vi "Parse VI XML - Splitter Size.vi"(8 "Is Vertical?":bool, 9 "UID":i32=83, 10 "New Size":i32, 11 "VI XML":string="<SL__rootObject class=\"oHExt\" uid=\"1\">\n  <root class=\"supC\" uid=\"10\">\n    <objFlags>65536</objFlags>\n    <bounds>(0, 0, 0, 0)</bounds>\n    <MouseWheelSupport>0</MouseWheelSupport>\n    <ddoList elements=\"1\">\n      <SL__arrayElement uid=\"206\"/>\n      </ddoList>\n    <paneHierarchy class=\"splitter\" uid=\"83\">\n      <objFlags>393232</objFlags>\n      <bounds>(46, 0, 434, 621)</bounds>\n      <partsList elements=\"3\">\n        <SL__arrayElement class=\"label\" uid=\"90\">\n          <objFlags>1511754</objFlags>\n          <partID>16</partID>\n          <masterPart>102</masterPart>\n          <howGrow>4108</howGrow>\n          <bounds>(133, 231, 255, 241)</bounds>\n          <image class=\"Image\">\n            <ImageResID>-9</ImageResID>\n            </image>\n          <fgColor>01000000</fgColor>\n          <bgColor>01000000</bgColor>\n          <textRec class=\"textHair\">\n            <mode>1029</mode>\n            <text>\"Splitter\"</text>\n            <bgColor>01000000</bgColor>\n            </textRec>\n          </SL__arrayElement>\n        <SL__arrayElement class=\"bigMultiCosm\" uid=\"91\">\n          <objFlags>2320</objFlags>\n          <partID>102</partID>\n          <bounds>(0, 228, 388, 234)</bounds>\n          <fgColor>00BCBCBC</fgColor>\n          <bgColor>00BCBCBC</bgColor>\n          <index>1</index>\n          <table elements=\"3\">\n            <SL__arrayElement class=\"SubCosm\">\n              <Bounds>(0, 0, 388, 6)</Bounds>\n              <FGColor>00BCBCBC</FGColor>\n              <BGColor>00BCBCBC</BGColor>\n              <Image class=\"Image\">\n                <ImageResID>-428</ImageResID>\n                </Image>\n              </SL__arrayElement>\n            <SL__arrayElement class=\"SubCosm\">\n              <Bounds>(0, 0, 388, 6)</Bounds>\n              <FGColor>00BCBCBC</FGColor>\n              <BGColor>00BCBCBC</BGColor>\n              <Image class=\"Image\">\n                <ImageResID>-11</ImageResID>\n                </Image>\n              </SL__arrayElement>\n            <SL__arrayElement class=\"SubCosm\">\n              <Bounds>(0, 0, 388, 6)</Bounds>\n              <FGColor>01000016</FGColor>\n              <BGColor>01000016</BGColor>\n              <Image class=\"Image\">\n                <ImageResID>-9</ImageResID>\n                </Image>\n              </SL__arrayElement>\n            </table>\n          </SL__arrayElement>\n        <SL__arrayElement class=\"annex\" uid=\"92\">\n          <partID>66</partID>\n          <refListLength>0</refListLength>\n          <hGrowNodeListLength>1</hGrowNodeListLength>\n          </SL__arrayElement>\n        </partsList>\n      <topOrLeft class=\"pane\" uid=\"104\">\n        <objFlags>2492464</objFlags>\n        <bounds>(0, 0, 388, 228)</bounds>\n        <partsList elements=\"6\">\n          <SL__arrayElement class=\"label\" uid=\"107\">\n            <objFlags>1511754</objFlags>\n            <partID>16</partID>\n            <masterPart>28</masterPart>\n            <howGrow>5</howGrow>\n            <bounds>(0, 0, 17, 29)</bounds>\n            <image class=\"Image\">\n              <ImageResID>-9</ImageResID>\n              </image>\n            <fgColor>01000000</fgColor>\n            <bgColor>01000000</bgColor>\n            <textRec class=\"textHair\">\n              <mode>1028</mode>\n              <text>\"Pane\"</text>\n              <bgColor>01000000</bgColor>\n              </textRec>\n            </SL__arrayElement>\n          <SL__arrayElement class=\"cosm\" uid=\"108\">\n            <objFlags>3442</objFlags>\n            <partID>39</partID>\n            <masterPart>28</masterPart>\n            <howGrow>194</howGrow>\n            <bounds>(0, 211, 371, 228)</bounds>\n            <image class=\"Image\">\n              <ImageResID>0</ImageResID>\n              </image>\n            <bgColor>00B3B3B3</bgColor>\n            </SL__arrayElement>\n          <SL__arrayElement class=\"cosm\" uid=\"109\">\n            <objFlags>3442</objFlags>\n            <partID>38</partID>\n            <masterPart>28</masterPart>\n            <howGrow>56</howGrow>\n            <bounds>(371, 0, 388, 211)</bounds>\n            <image class=\"Image\">\n              <ImageResID>0</ImageResID>\n              </image>\n            <bgColor>00B3B3B3</bgColor>\n            </SL__arrayElement>\n          <SL__arrayElement class=\"cosm\" uid=\"110\">\n            <objFlags>3443</objFlags>\n            <partID>44</partID>\n            <masterPart>28</masterPart>\n            <howGrow>10</howGrow>\n            <bounds>(371, 211, 388, 228)</bounds>\n            <image class=\"Image\">\n              <ImageResID>-365</ImageResID>\n              </image>\n            <fgColor>00B3B3B3</fgColor>\n            <bgColor>00B3B3B3</bgColor>\n            </SL__arrayElement>\n          <SL__arrayElement class=\"cosm\" uid=\"111\">\n            <objFlags>115</objFlags>\n            <partID>28</partID>\n            <howGrow>120</howGrow>\n            <bounds>(0, 0, 371, 211)</bounds>\n            <image class=\"Image\">\n              <ImageResID>-704</ImageResID>\n              </image>\n            <fgColor>00E2E2E2</fgColor>\n            <bgColor>00E2E2E2</bgColor>\n            </SL__arrayElement>\n          <SL__arrayElement class=\"annex\" uid=\"112\">\n            <partID>66</partID>\n            </SL__arrayElement>\n          </partsList>\n        <paneFlags>331089</paneFlags>\n        <minPaneSize>(1,1)</minPaneSize>\n        <docBounds>(-138, 0, 325, 232)</docBounds>\n        <zPlaneList elements=\"1\">\n          <SL__arrayElement class=\"fPDCO\" uid=\"206\">\n            <objFlags>1</objFlags>\n            <typeDesc>TypeID(1)</typeDesc>\n            <ddo class=\"stdNum\" uid=\"190\">\n              <objFlags>393217</objFlags>\n              <bounds>(0, 105, 41, 180)</bounds>\n              <partsList elements=\"8\">\n                <SL__arrayElement class=\"label\" uid=\"196\">\n                  <objFlags>1507654</objFlags>\n                  <partID>16</partID>\n                  <masterPart>9</masterPart>\n                  <howGrow>4096</howGrow>\n                  <bounds>(0, 0, 17, 22)</bounds>\n                  <image class=\"Image\">\n                    <ImageResID>-9</ImageResID>\n                    </image>\n                  <fgColor>01000000</fgColor>\n                  <bgColor>01000000</bgColor>\n                  <textRec class=\"textHair\">\n                    <flags>512</flags>\n                    <mode>17412</mode>\n                    <text>\"UID\"</text>\n                    <bgColor>01000000</bgColor>\n                    </textRec>\n                  </SL__arrayElement>\n                <SL__arrayElement class=\"numLabel\" uid=\"197\">\n                  <objFlags>264498</objFlags>\n                  <partID>10</partID>\n                  <masterPart>9</masterPart>\n                  <howGrow>240</howGrow>\n                  <bounds>(19, 2, 39, 74)</bounds>\n                  <image class=\"Image\">\n                    <ImageResID>-2002</ImageResID>\n                    </image>\n                  <fgColor>00FFFFFF</fgColor>\n                  <bgColor>00E8EBED</bgColor>\n                  <textRec class=\"textHair\">\n                    <flags>1536</flags>\n                    <mode>8389650</mode>\n                    <view>(1, 0, -2, 0)</view>\n                    <bgColor>00E8EBED</bgColor>\n                    </textRec>\n                  <format>\"%25.0f\"</format>\n                  </SL__arrayElement>\n                <SL__arrayElement class=\"bigMultiCosm\" uid=\"198\">\n                  <objFlags>6458</objFlags>\n                  <partID>2</partID>\n                  <masterPart>9</masterPart>\n                  <howGrow>2054</howGrow>\n                  <bounds>(17, 62, 28, 75)</bounds>\n                  <fgColor>002B3033</fgColor>\n                  <bgColor>00A8ABAE</bgColor>\n                  <table elements=\"2\">\n                    <SL__arrayElement class=\"SubCosm\">\n                      <Bounds>(0, 0, 11, 13)</Bounds>\n                      <FGColor>002B3033</FGColor>\n                      <BGColor>00A8ABAE</BGColor>\n                      <Image class=\"Image\">\n                        <ImageResID>-774</ImageResID>\n                        </Image>\n                      </SL__arrayElement>\n                    <SL__arrayElement class=\"SubCosm\">\n                      <Bounds>(0, 0, 11, 13)</Bounds>\n                      <FGColor>002B3033</FGColor>\n                      <BGColor>004384B7</BGColor>\n                      <Image class=\"Image\">\n                        <ImageResID>-774</ImageResID>\n                        </Image>\n                      </SL__arrayElement>\n                    </table>\n                  </SL__arrayElement>\n                <SL__arrayElement class=\"bigMultiCosm\" uid=\"199\">\n                  <objFlags>6458</objFlags>\n                  <partID>3</partID>\n                  <masterPart>9</masterPart>\n                  <howGrow>1034</howGrow>\n                  <bounds>(30, 62, 41, 75)</bounds>\n                  <fgColor>002B3033</fgColor>\n                  <bgColor>00A8ABAE</bgColor>\n                  <table elements=\"2\">\n                    <SL__arrayElement class=\"SubCosm\">\n                      <Bounds>(0, 0, 11, 13)</Bounds>\n                      <FGColor>002B3033</FGColor>\n                      <BGColor>00A8ABAE</BGColor>\n                      <Image class=\"Image\">\n                        <ImageResID>-775</ImageResID>\n                        </Image>\n                      </SL__arrayElement>\n                    <SL__arrayElement class=\"SubCosm\">\n                      <Bounds>(0, 0, 11, 13)</Bounds>\n                      <FGColor>002B3033</FGColor>\n                      <BGColor>004384B7</BGColor>\n                      <Image class=\"Image\">\n                        <ImageResID>-775</ImageResID>\n                        </Image>\n                      </SL__arrayElement>\n                    </table>\n                  </SL__arrayElement>\n                <SL__arrayElement class=\"multiCosm\" uid=\"200\">\n                  <objFlags>6458</objFlags>\n                  <partID>15</partID>\n                  <masterPart>9</masterPart>\n                  <howGrow>13</howGrow>\n                  <bounds>(22, 1, 37, 7)</bounds>\n                  <fgColor>002B3033</fgColor>\n                  <bgColor>00DBDFE2</bgColor>\n                  <table elements=\"5\">\n                    <SL__arrayElement class=\"Image\">\n                      <ImageResID>-2000</ImageResID>\n                      </SL__arrayElement>\n                    <SL__arrayElement class=\"Image\">\n                      <ImageResID>-2001</ImageResID>\n                      </SL__arrayElement>\n                    <SL__arrayElement class=\"Image\">\n                      <ImageResID>-2002</ImageResID>\n                      </SL__arrayElement>\n                    <SL__arrayElement class=\"Image\">\n                      <ImageResID>-2003</ImageResID>\n                      </SL__arrayElement>\n                    <SL__arrayElement class=\"Image\">\n                      <ImageResID>-2095</ImageResID>\n                      </SL__arrayElement>\n                    </table>\n                  </SL__arrayElement>\n                <SL__arrayElement class=\"multiCosm\" uid=\"201\">\n                  <objFlags>6462</objFlags>\n                  <partID>118</partID>\n                  <masterPart>9</masterPart>\n                  <howGrow>193</howGrow>\n                  <bounds>(18, 1, 40, 7)</bounds>\n                  <fgColor>00DBDFE2</fgColor>\n                  <bgColor>00DBDFE2</bgColor>\n                  <table elements=\"5\">\n                    <SL__arrayElement class=\"Image\">\n                      <ImageResID>-11</ImageResID>\n                      </SL__arrayElement>\n                    <SL__arrayElement class=\"Image\">\n                      <ImageResID>-11</ImageResID>\n                      </SL__arrayElement>\n                    <SL__arrayElement class=\"Image\">\n                      <ImageResID>-11</ImageResID>\n                      </SL__arrayElement>\n                    <SL__arrayElement class=\"Image\">\n                      <ImageResID>-11</ImageResID>\n                      </SL__arrayElement>\n                    <SL__arrayElement class=\"Image\">\n                      <ImageResID>-11</ImageResID>\n                      </SL__arrayElement>\n                    </table>\n                  </SL__arrayElement>\n                <SL__arrayElement class=\"cosm\" uid=\"202\">\n                  <objFlags>2327</objFlags>\n                  <partID>9</partID>\n                  <howGrow>240</howGrow>\n                  <bounds>(17, 0, 41, 75)</bounds>\n                  <image class=\"Image\">\n                    <ImageResID>-786</ImageResID>\n                    </image>\n                  <fgColor>00A8ABAE</fgColor>\n                  <bgColor>00E8EBED</bgColor>\n                  </SL__arrayElement>\n                <SL__arrayElement class=\"annex\" uid=\"203\">\n                  <partID>66</partID>\n                  <refListLength>0</refListLength>\n                  <hGrowNodeListLength>0</hGrowNodeListLength>\n                  <rsrcID>32707</rsrcID>\n                  </SL__arrayElement>\n                </partsList>\n              <typeDesc>TypeID(2)</typeDesc>\n              <MouseWheelSupport>2</MouseWheelSupport>\n              <StdNumMin>-2147483648</StdNumMin>\n              <StdNumMax>2147483647</StdNumMax>\n              <StdNumInc>0</StdNumInc>\n              </ddo>\n            <conNum>-1</conNum>\n            <termListLength>1</termListLength>\n            </SL__arrayElement>\n          </zPlaneList>\n        <image class=\"Image\">\n          <ImageResID>0</ImageResID>\n          </image>\n        </topOrLeft>\n      <botOrRight class=\"pane\" uid=\"95\">\n        <objFlags>2492464</objFlags>\n        <bounds>(0, 234, 388, 621)</bounds>\n        <partsList elements=\"6\">\n          <SL__arrayElement class=\"label\" uid=\"98\">\n            <objFlags>1511754</objFlags>\n            <partID>16</partID>\n            <masterPart>28</masterPart>\n            <howGrow>5</howGrow>\n            <bounds>(0, 0, 17, 38)</bounds>\n            <image class=\"Image\">\n              <ImageResID>-9</ImageResID>\n              </image>\n            <fgColor>01000000</fgColor>\n            <bgColor>01000000</bgColor>\n            <textRec class=\"textHair\">\n              <mode>1028</mode>\n              <text>\"Pane 2\"</text>\n              <bgColor>01000000</bgColor>\n              </textRec>\n            </SL__arrayElement>\n          <SL__arrayElement class=\"cosm\" uid=\"99\">\n            <objFlags>3442</objFlags>\n            <partID>39</partID>\n            <masterPart>28</masterPart>\n            <howGrow>194</howGrow>\n            <bounds>(0, 370, 371, 387)</bounds>\n            <image class=\"Image\">\n              <ImageResID>0</ImageResID>\n              </image>\n            <bgColor>00B3B3B3</bgColor>\n            </SL__arrayElement>\n          <SL__arrayElement class=\"cosm\" uid=\"100\">\n            <objFlags>3442</objFlags>\n            <partID>38</partID>\n            <masterPart>28</masterPart>\n            <howGrow>56</howGrow>\n            <bounds>(371, 0, 388, 370)</bounds>\n            <image class=\"Image\">\n              <ImageResID>0</ImageResID>\n              </image>\n            <bgColor>00B3B3B3</bgColor>\n            </SL__arrayElement>\n          <SL__arrayElement class=\"cosm\" uid=\"101\">\n            <objFlags>3443</objFlags>\n            <partID>44</partID>\n            <masterPart>28</masterPart>\n            <howGrow>10</howGrow>\n            <bounds>(371, 370, 388, 387)</bounds>\n            <image class=\"Image\">\n              <ImageResID>-365</ImageResID>\n              </image>\n            <fgColor>00B3B3B3</fgColor>\n            <bgColor>00B3B3B3</bgColor>\n            </SL__arrayElement>\n          <SL__arrayElement class=\"cosm\" uid=\"102\">\n            <objFlags>115</objFlags>\n            <partID>28</partID>\n            <howGrow>120</howGrow>\n            <bounds>(0, 0, 371, 370)</bounds>\n            <image class=\"Image\">\n              <ImageResID>-704</ImageResID>\n              </image>\n            <fgColor>00E2E2E2</fgColor>\n            <bgColor>00E2E2E2</bgColor>\n            </SL__arrayElement>\n          <SL__arrayElement class=\"annex\" uid=\"103\">\n            <partID>66</partID>\n            </SL__arrayElement>\n          </partsList>\n        <paneFlags>331089</paneFlags>\n        <minPaneSize>(1,1)</minPaneSize>\n        <docBounds>(-46, 0, 325, 370)</docBounds>\n        <zPlaneList elements=\"0\">\n          </zPlaneList>\n        <image class=\"Image\">\n          <ImageResID>0</ImageResID>\n          </image>\n        </botOrRight>\n      <splitterFlags>1</splitterFlags>\n      <ratio>3.671498E-1 (%x0EFBBB3E)</ratio>\n      </paneHierarchy>\n    <savedSize>(0, 0, 0, 0)</savedSize>\n    <conPane class=\"conPane\" uid=\"21\">\n      <conId>4815</conId>\n      <cons elements=\"12\">\n        </cons>\n      </conPane>\n    <keyMappingList class=\"keyMapList\" uid=\"22\">\n      </keyMappingList>\n    </root>\n  <pBounds>(46, 0, 434, 621)</pBounds>\n  <dBounds>(0, 0, 0, 0)</dBounds>\n  <origin>(435,189)</origin>\n  <instrStyle>31</instrStyle>\n  <blinkList elements=\"0\">\n    </blinkList>\n  </SL__rootObject>\n") -> (2 "Old Size":i32, 3 "VI XML With New Size":string="<SL__rootObject class=\"oHExt\" uid=\"1\">\n  <root class=\"supC\" uid=\"10\">\n    <objFlags>65536</objFlags>\n    <bounds>(0, 0, 0, 0)</bounds>\n    <MouseWheelSupport>0</MouseWheelSupport>\n    <ddoList elements=\"1\">\n      <SL__arrayElement uid=\"206\"/>\n      </ddoList>\n    <paneHierarchy class=\"splitter\" uid=\"83\">\n      <objFlags>393232</objFlags>\n      <bounds>(46, 0, 434, 621)</bounds>\n      <partsList elements=\"3\">\n        <SL__arrayElement class=\"label\" uid=\"90\">\n          <objFlags>1511754</objFlags>\n          <partID>16</partID>\n          <masterPart>102</masterPart>\n          <howGrow>4108</howGrow>\n          <bounds>(133, 231, 255, 241)</bounds>\n          <image class=\"Image\">\n            <ImageResID>-9</ImageResID>\n            </image>\n          <fgColor>01000000</fgColor>\n          <bgColor>01000000</bgColor>\n          <textRec class=\"textHair\">\n            <mode>1029</mode>\n            <text>\"Splitter\"</text>\n            <bgColor>01000000</bgColor>\n            </textRec>\n          </SL__arrayElement>\n        <SL__arrayElement class=\"bigMultiCosm\" uid=\"91\">\n          <objFlags>2320</objFlags>\n          <partID>102</partID>\n          <bounds>(0, 228, 388, 234)</bounds>\n          <fgColor>00BCBCBC</fgColor>\n          <bgColor>00BCBCBC</bgColor>\n          <index>1</index>\n          <table elements=\"3\">\n            <SL__arrayElement class=\"SubCosm\">\n              <Bounds>(0, 0, 388, 6)</Bounds>\n              <FGColor>00BCBCBC</FGColor>\n              <BGColor>00BCBCBC</BGColor>\n              <Image class=\"Image\">\n                <ImageResID>-428</ImageResID>\n                </Image>\n              </SL__arrayElement>\n            <SL__arrayElement class=\"SubCosm\">\n              <Bounds>(0, 0, 388, 6)</Bounds>\n              <FGColor>00BCBCBC</FGColor>\n              <BGColor>00BCBCBC</BGColor>\n              <Image class=\"Image\">\n                <ImageResID>-11</ImageResID>\n                </Image>\n              </SL__arrayElement>\n            <SL__arrayElement class=\"SubCosm\">\n              <Bounds>(0, 0, 388, 6)</Bounds>\n              <FGColor>01000016</FGColor>\n              <BGColor>01000016</BGColor>\n              <Image class=\"Image\">\n                <ImageResID>-9</ImageResID>\n                </Image>\n              </SL__arrayElement>\n            </table>\n          </SL__arrayElement>\n        <SL__arrayElement class=\"annex\" uid=\"92\">\n          <partID>66</partID>\n          <refListLength>0</refListLength>\n          <hGrowNodeListLength>1</hGrowNodeListLength>\n          </SL__arrayElement>\n        </partsList>\n      <topOrLeft class=\"pane\" uid=\"104\">\n        <objFlags>2492464</objFlags>\n        <bounds>(0, 0, 388, 228)</bounds>\n        <partsList elements=\"6\">\n          <SL__arrayElement class=\"label\" uid=\"107\">\n            <objFlags>1511754</objFlags>\n            <partID>16</partID>\n            <masterPart>28</masterPart>\n            <howGrow>5</howGrow>\n            <bounds>(0, 0, 17, 29)</bounds>\n            <image class=\"Image\">\n              <ImageResID>-9</ImageResID>\n              </image>\n            <fgColor>01000000</fgColor>\n            <bgColor>01000000</bgColor>\n            <textRec class=\"textHair\">\n              <mode>1028</mode>\n              <text>\"Pane\"</text>\n              <bgColor>01000000</bgColor>\n              </textRec>\n            </SL__arrayElement>\n          <SL__arrayElement class=\"cosm\" uid=\"108\">\n            <objFlags>3442</objFlags>\n            <partID>39</partID>\n            <masterPart>28</masterPart>\n            <howGrow>194</howGrow>\n            <bounds>(0, 211, 371, 228)</bounds>\n            <image class=\"Image\">\n              <ImageResID>0</ImageResID>\n              </image>\n            <bgColor>00B3B3B3</bgColor>\n            </SL__arrayElement>\n          <SL__arrayElement class=\"cosm\" uid=\"109\">\n            <objFlags>3442</objFlags>\n            <partID>38</partID>\n            <masterPart>28</masterPart>\n            <howGrow>56</howGrow>\n            <bounds>(371, 0, 388, 211)</bounds>\n            <image class=\"Image\">\n              <ImageResID>0</ImageResID>\n              </image>\n            <bgColor>00B3B3B3</bgColor>\n            </SL__arrayElement>\n          <SL__arrayElement class=\"cosm\" uid=\"110\">\n            <objFlags>3443</objFlags>\n            <partID>44</partID>\n            <masterPart>28</masterPart>\n            <howGrow>10</howGrow>\n            <bounds>(371, 211, 388, 228)</bounds>\n            <image class=\"Image\">\n              <ImageResID>-365</ImageResID>\n              </image>\n            <fgColor>00B3B3B3</fgColor>\n            <bgColor>00B3B3B3</bgColor>\n            </SL__arrayElement>\n          <SL__arrayElement class=\"cosm\" uid=\"111\">\n            <objFlags>115</objFlags>\n            <partID>28</partID>\n            <howGrow>120</howGrow>\n            <bounds>(0, 0, 371, 211)</bounds>\n            <image class=\"Image\">\n              <ImageResID>-704</ImageResID>\n              </image>\n            <fgColor>00E2E2E2</fgColor>\n            <bgColor>00E2E2E2</bgColor>\n            </SL__arrayElement>\n          <SL__arrayElement class=\"annex\" uid=\"112\">\n            <partID>66</partID>\n            </SL__arrayElement>\n          </partsList>\n        <paneFlags>331089</paneFlags>\n        <minPaneSize>(1,1)</minPaneSize>\n        <docBounds>(-138, 0, 325, 232)</docBounds>\n        <zPlaneList elements=\"1\">\n          <SL__arrayElement class=\"fPDCO\" uid=\"206\">\n            <objFlags>1</objFlags>\n            <typeDesc>TypeID(1)</typeDesc>\n            <ddo class=\"stdNum\" uid=\"190\">\n              <objFlags>393217</objFlags>\n              <bounds>(0, 105, 41, 180)</bounds>\n              <partsList elements=\"8\">\n                <SL__arrayElement class=\"label\" uid=\"196\">\n                  <objFlags>1507654</objFlags>\n                  <partID>16</partID>\n                  <masterPart>9</masterPart>\n                  <howGrow>4096</howGrow>\n                  <bounds>(0, 0, 17, 22)</bounds>\n                  <image class=\"Image\">\n                    <ImageResID>-9</ImageResID>\n                    </image>\n                  <fgColor>01000000</fgColor>\n                  <bgColor>01000000</bgColor>\n                  <textRec class=\"textHair\">\n                    <flags>512</flags>\n                    <mode>17412</mode>\n                    <text>\"UID\"</text>\n                    <bgColor>01000000</bgColor>\n                    </textRec>\n                  </SL__arrayElement>\n                <SL__arrayElement class=\"numLabel\" uid=\"197\">\n                  <objFlags>264498</objFlags>\n                  <partID>10</partID>\n                  <masterPart>9</masterPart>\n                  <howGrow>240</howGrow>\n                  <bounds>(19, 2, 39, 74)</bounds>\n                  <image class=\"Image\">\n                    <ImageResID>-2002</ImageResID>\n                    </image>\n                  <fgColor>00FFFFFF</fgColor>\n                  <bgColor>00E8EBED</bgColor>\n                  <textRec class=\"textHair\">\n                    <flags>1536</flags>\n                    <mode>8389650</mode>\n                    <view>(1, 0, -2, 0)</view>\n                    <bgColor>00E8EBED</bgColor>\n                    </textRec>\n                  <format>\"%25.0f\"</format>\n                  </SL__arrayElement>\n                <SL__arrayElement class=\"bigMultiCosm\" uid=\"198\">\n                  <objFlags>6458</objFlags>\n                  <partID>2</partID>\n                  <masterPart>9</masterPart>\n                  <howGrow>2054</howGrow>\n                  <bounds>(17, 62, 28, 75)</bounds>\n                  <fgColor>002B3033</fgColor>\n                  <bgColor>00A8ABAE</bgColor>\n                  <table elements=\"2\">\n                    <SL__arrayElement class=\"SubCosm\">\n                      <Bounds>(0, 0, 11, 13)</Bounds>\n                      <FGColor>002B3033</FGColor>\n                      <BGColor>00A8ABAE</BGColor>\n                      <Image class=\"Image\">\n                        <ImageResID>-774</ImageResID>\n                        </Image>\n                      </SL__arrayElement>\n                    <SL__arrayElement class=\"SubCosm\">\n                      <Bounds>(0, 0, 11, 13)</Bounds>\n                      <FGColor>002B3033</FGColor>\n                      <BGColor>004384B7</BGColor>\n                      <Image class=\"Image\">\n                        <ImageResID>-774</ImageResID>\n                        </Image>\n                      </SL__arrayElement>\n                    </table>\n                  </SL__arrayElement>\n                <SL__arrayElement class=\"bigMultiCosm\" uid=\"199\">\n                  <objFlags>6458</objFlags>\n                  <partID>3</partID>\n                  <masterPart>9</masterPart>\n                  <howGrow>1034</howGrow>\n                  <bounds>(30, 62, 41, 75)</bounds>\n                  <fgColor>002B3033</fgColor>\n                  <bgColor>00A8ABAE</bgColor>\n                  <table elements=\"2\">\n                    <SL__arrayElement class=\"SubCosm\">\n                      <Bounds>(0, 0, 11, 13)</Bounds>\n                      <FGColor>002B3033</FGColor>\n                      <BGColor>00A8ABAE</BGColor>\n                      <Image class=\"Image\">\n                        <ImageResID>-775</ImageResID>\n                        </Image>\n                      </SL__arrayElement>\n                    <SL__arrayElement class=\"SubCosm\">\n                      <Bounds>(0, 0, 11, 13)</Bounds>\n                      <FGColor>002B3033</FGColor>\n                      <BGColor>004384B7</BGColor>\n                      <Image class=\"Image\">\n                        <ImageResID>-775</ImageResID>\n                        </Image>\n                      </SL__arrayElement>\n                    </table>\n                  </SL__arrayElement>\n                <SL__arrayElement class=\"multiCosm\" uid=\"200\">\n                  <objFlags>6458</objFlags>\n                  <partID>15</partID>\n                  <masterPart>9</masterPart>\n                  <howGrow>13</howGrow>\n                  <bounds>(22, 1, 37, 7)</bounds>\n                  <fgColor>002B3033</fgColor>\n                  <bgColor>00DBDFE2</bgColor>\n                  <table elements=\"5\">\n                    <SL__arrayElement class=\"Image\">\n                      <ImageResID>-2000</ImageResID>\n                      </SL__arrayElement>\n                    <SL__arrayElement class=\"Image\">\n                      <ImageResID>-2001</ImageResID>\n                      </SL__arrayElement>\n                    <SL__arrayElement class=\"Image\">\n                      <ImageResID>-2002</ImageResID>\n                      </SL__arrayElement>\n                    <SL__arrayElement class=\"Image\">\n                      <ImageResID>-2003</ImageResID>\n                      </SL__arrayElement>\n                    <SL__arrayElement class=\"Image\">\n                      <ImageResID>-2095</ImageResID>\n                      </SL__arrayElement>\n                    </table>\n                  </SL__arrayElement>\n                <SL__arrayElement class=\"multiCosm\" uid=\"201\">\n                  <objFlags>6462</objFlags>\n                  <partID>118</partID>\n                  <masterPart>9</masterPart>\n                  <howGrow>193</howGrow>\n                  <bounds>(18, 1, 40, 7)</bounds>\n                  <fgColor>00DBDFE2</fgColor>\n                  <bgColor>00DBDFE2</bgColor>\n                  <table elements=\"5\">\n                    <SL__arrayElement class=\"Image\">\n                      <ImageResID>-11</ImageResID>\n                      </SL__arrayElement>\n                    <SL__arrayElement class=\"Image\">\n                      <ImageResID>-11</ImageResID>\n                      </SL__arrayElement>\n                    <SL__arrayElement class=\"Image\">\n                      <ImageResID>-11</ImageResID>\n                      </SL__arrayElement>\n                    <SL__arrayElement class=\"Image\">\n                      <ImageResID>-11</ImageResID>\n                      </SL__arrayElement>\n                    <SL__arrayElement class=\"Image\">\n                      <ImageResID>-11</ImageResID>\n                      </SL__arrayElement>\n                    </table>\n                  </SL__arrayElement>\n                <SL__arrayElement class=\"cosm\" uid=\"202\">\n                  <objFlags>2327</objFlags>\n                  <partID>9</partID>\n                  <howGrow>240</howGrow>\n                  <bounds>(17, 0, 41, 75)</bounds>\n                  <image class=\"Image\">\n                    <ImageResID>-786</ImageResID>\n                    </image>\n                  <fgColor>00A8ABAE</fgColor>\n                  <bgColor>00E8EBED</bgColor>\n                  </SL__arrayElement>\n                <SL__arrayElement class=\"annex\" uid=\"203\">\n                  <partID>66</partID>\n                  <refListLength>0</refListLength>\n                  <hGrowNodeListLength>0</hGrowNodeListLength>\n                  <rsrcID>32707</rsrcID>\n                  </SL__arrayElement>\n                </partsList>\n              <typeDesc>TypeID(2)</typeDesc>\n              <MouseWheelSupport>2</MouseWheelSupport>\n              <StdNumMin>-2147483648</StdNumMin>\n              <StdNumMax>2147483647</StdNumMax>\n              <StdNumInc>0</StdNumInc>\n              </ddo>\n            <conNum>-1</conNum>\n            <termListLength>1</termListLength>\n            </SL__arrayElement>\n          </zPlaneList>\n        <image class=\"Image\">\n          <ImageResID>0</ImageResID>\n          </image>\n        </topOrLeft>\n      <botOrRight class=\"pane\" uid=\"95\">\n        <objFlags>2492464</objFlags>\n        <bounds>(0, 234, 388, 621)</bounds>\n        <partsList elements=\"6\">\n          <SL__arrayElement class=\"label\" uid=\"98\">\n            <objFlags>1511754</objFlags>\n            <partID>16</partID>\n            <masterPart>28</masterPart>\n            <howGrow>5</howGrow>\n            <bounds>(0, 0, 17, 38)</bounds>\n            <image class=\"Image\">\n              <ImageResID>-9</ImageResID>\n              </image>\n            <fgColor>01000000</fgColor>\n            <bgColor>01000000</bgColor>\n            <textRec class=\"textHair\">\n              <mode>1028</mode>\n              <text>\"Pane 2\"</text>\n              <bgColor>01000000</bgColor>\n              </textRec>\n            </SL__arrayElement>\n          <SL__arrayElement class=\"cosm\" uid=\"99\">\n            <objFlags>3442</objFlags>\n            <partID>39</partID>\n            <masterPart>28</masterPart>\n            <howGrow>194</howGrow>\n            <bounds>(0, 370, 371, 387)</bounds>\n            <image class=\"Image\">\n              <ImageResID>0</ImageResID>\n              </image>\n            <bgColor>00B3B3B3</bgColor>\n            </SL__arrayElement>\n          <SL__arrayElement class=\"cosm\" uid=\"100\">\n            <objFlags>3442</objFlags>\n            <partID>38</partID>\n            <masterPart>28</masterPart>\n            <howGrow>56</howGrow>\n            <bounds>(371, 0, 388, 370)</bounds>\n            <image class=\"Image\">\n              <ImageResID>0</ImageResID>\n              </image>\n            <bgColor>00B3B3B3</bgColor>\n            </SL__arrayElement>\n          <SL__arrayElement class=\"cosm\" uid=\"101\">\n            <objFlags>3443</objFlags>\n            <partID>44</partID>\n            <masterPart>28</masterPart>\n            <howGrow>10</howGrow>\n            <bounds>(371, 370, 388, 387)</bounds>\n            <image class=\"Image\">\n              <ImageResID>-365</ImageResID>\n              </image>\n            <fgColor>00B3B3B3</fgColor>\n            <bgColor>00B3B3B3</bgColor>\n            </SL__arrayElement>\n          <SL__arrayElement class=\"cosm\" uid=\"102\">\n            <objFlags>115</objFlags>\n            <partID>28</partID>\n            <howGrow>120</howGrow>\n            <bounds>(0, 0, 371, 370)</bounds>\n            <image class=\"Image\">\n              <ImageResID>-704</ImageResID>\n              </image>\n            <fgColor>00E2E2E2</fgColor>\n            <bgColor>00E2E2E2</bgColor>\n            </SL__arrayElement>\n          <SL__arrayElement class=\"annex\" uid=\"103\">\n            <partID>66</partID>\n            </SL__arrayElement>\n          </partsList>\n        <paneFlags>331089</paneFlags>\n        <minPaneSize>(1,1)</minPaneSize>\n        <docBounds>(-46, 0, 325, 370)</docBounds>\n        <zPlaneList elements=\"0\">\n          </zPlaneList>\n        <image class=\"Image\">\n          <ImageResID>0</ImageResID>\n          </image>\n        </botOrRight>\n      <splitterFlags>1</splitterFlags>\n      <ratio>3.671498E-1 (%x0EFBBB3E)</ratio>\n      </paneHierarchy>\n    <savedSize>(0, 0, 0, 0)</savedSize>\n    <conPane class=\"conPane\" uid=\"21\">\n      <conId>4815</conId>\n      <cons elements=\"12\">\n        </cons>\n      </conPane>\n    <keyMappingList class=\"keyMapList\" uid=\"22\">\n      </keyMappingList>\n    </root>\n  <pBounds>(46, 0, 434, 621)</pBounds>\n  <dBounds>(0, 0, 0, 0)</dBounds>\n  <origin>(435,189)</origin>\n  <instrStyle>31</instrStyle>\n  <blinkList elements=\"0\">\n    </blinkList>\n  </SL__rootObject>\n")   [LabVIEW 2015, in "Splitter.lvclass"]
uses:
  Splitter.lvclass
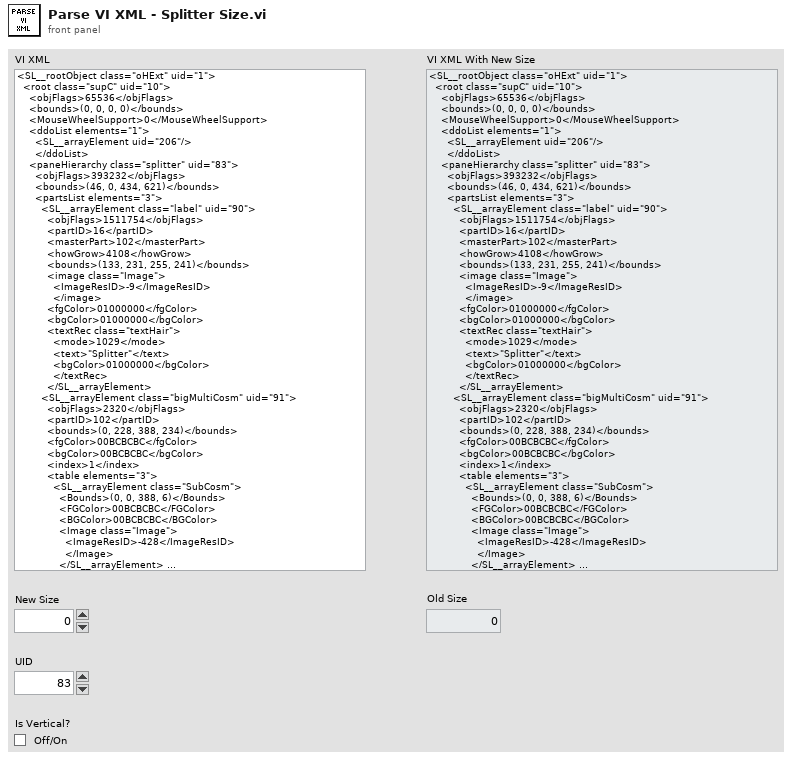
[diagram p1: front panel]
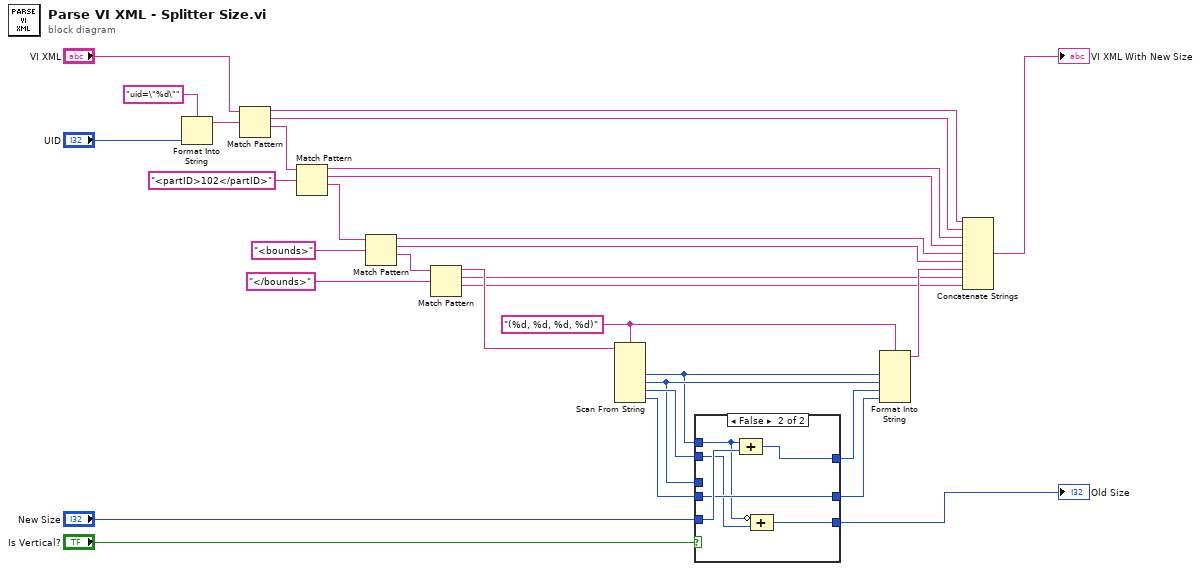
[diagram p0: block diagram]
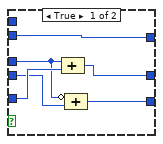
[diagram p2: hidden frame]
diagram:
  w21 = "(%d, %d, %d, %d)" ("format string")
  n1 = Format Into String(format string="uid=\"%d\"", "UID") -> (resulting string=w30:string)  [unwired: 2 in, 1 out]
  n2 = Match Pattern(string="VI XML", regular expression=w30) -> (before substring=w12:string, match substring=w13:string, after substring=w28:string)  [unwired: 1 in, 1 out]
  n3 = Match Pattern(string=w28, regular expression="<partID>102</partID>" ("format string")) -> (before substring=w14:string, match substring=w15:string, after substring=w26:string)  [unwired: 1 in, 1 out]
  n4 = Match Pattern(string=w26, regular expression="<bounds>" ("format string")) -> (before substring=w16:string, match substring=w17:string, after substring=w24:string)  [unwired: 1 in, 1 out]
  n5 = Match Pattern(string=w24, regular expression="</bounds>" ("format string")) -> (before substring=w22:string, match substring=w19:string, after substring=w18:string)  [unwired: 1 in, 1 out]
  n6 = Scan From String(format string=w21, input string=w22) -> (output 1=w4:i32, output 2=w6:i32, output 3=w8:i32, output 4=w7:i32)  [unwired: 6 in, 3 out]
  n7 = case shown="False" "Is Vertical?" {
    tunnel: [w35 w42] -> w3
    tunnel: w8 -> [w35 w38]
    tunnel: [w36 w41] -> w2
    tunnel: w7 -> [w34 w41]
    tunnel: w6 -> [w32 _]
    tunnel: "New Size" -> [w37 w43]
    tunnel: w4 -> [_ w40]
    tunnel: [w33 w39] -> w1
    frame True {
      n8 = Compound Arithmetic op=ADD(w32, w37) -> (w36:i32)
      n9 = Compound Arithmetic op=ADD(invert w32, w34) -> (w33:i32)
    }
    frame False {
      n10 = Compound Arithmetic op=ADD(w40, w43) -> (w42:i32)
      n11 = Compound Arithmetic op=ADD(invert w40, w38) -> (w39:i32)
    }
  }
  "Old Size" <- w1
  n12 = Format Into String(format string=w21, w4, w6, w3, w2) -> (resulting string=w20:string)  [unwired: 2 in, 1 out]
  n13 = Concatenate Strings(w12, w13, w14, w15, w16, w17, w20, w19, w18) -> (→"VI XML With New Size":string)
